vi "trackingNotification_Create.vi"(8 "error in (no error)":errorcluster, 9 "dim":i32, 10 "index":i32, 11 "reference in":refnum<class "trackingNotification.lvclass">) -> (0 "error out":errorcluster, 3 "reference out":refnum<class "trackingNotification.lvclass">)   [LabVIEW 2015, in "trackingNotification.lvclass"]
doc: "Constructor."
uses:
  trackingNotification.lvclass
  <vilib>/addons/_AddQ/G#Object/utils/G#Object_CreateMethod.ctl
  <vilib>/addons/_AddQ/G#Object/G#Object.lvclass
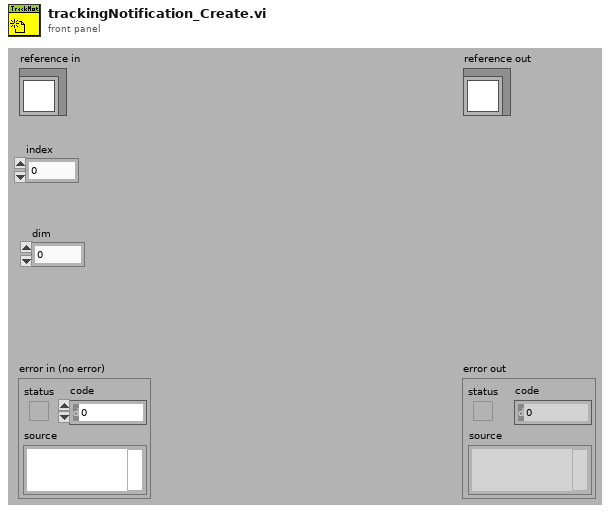
[diagram p1: front panel]
types:
  T1 = typedef "G#Object.lvclass/G#Object_CreateMethod.ctl" = enum16{"Create", "Create or look up existing", "Look up existing"}
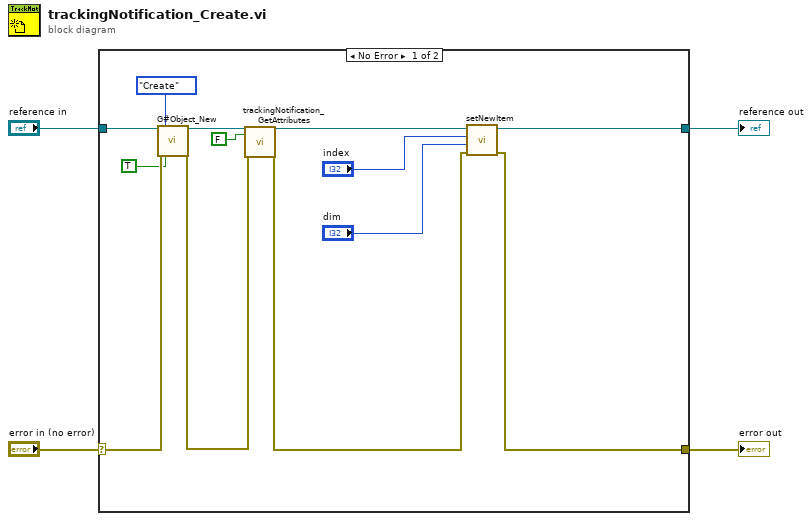
[diagram p0: block diagram]
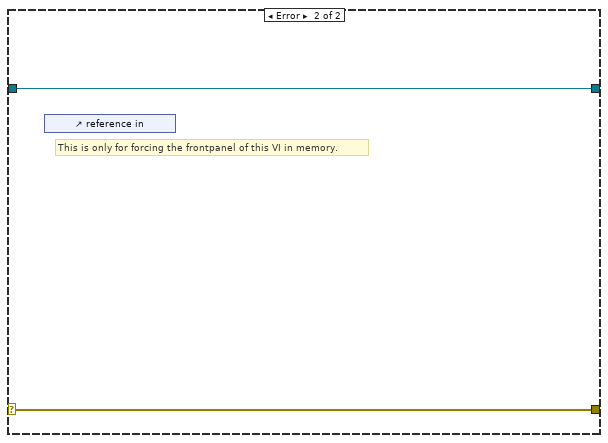
[diagram p2: hidden frame]
diagram:
  n1 = case shown="No Error" "error in (no error)" {
    selector: "error in (no error)" -> [w16 w19]
    tunnel: [w9 w19] -> w3
    tunnel: [w7 w18] -> w1
    tunnel: "reference in" -> [w17 w18]
    frame No Error {
      n2 = call <vilib>:"G#Object_New.vi"("reference in"=w17, "error in (no error)"=w16, "create method"=G#Object_CreateMethod."Create", "user counter (T)?"=TRUE ("User Counter")) -> ("reference out"=w14:refnum<class "trackingNotification.lvclass">, "error out"=w13:errorcluster)  [unwired: 13 in, 1 out]
      n3 = call "trackingNotification_GetAttributes.vi"("reference in"=w14, "return data? (T)"=FALSE ("return data"), "error in (no error)"=w13) -> ("reference out"=w8:refnum<class "trackingNotification.lvclass">, "error out"=w10:errorcluster)  [unwired: 13 in, 2 out]
      n4 = call "setNewItem.vi"("error in (no error)"=w10, "dim"="dim", "index"="index", "reference in"=w8) -> ("error out"=w9:errorcluster, "reference out"=w7:refnum<class "trackingNotification.lvclass">)  [unwired: 6 in]
    }
    frame Error {
      # "This is only for forcing the frontpanel of this VI in memory."
      n5 = control-ref of="reference in"() -> ()  [unwired: 1 out]
    }
  }
  "error out" <- w3
  "reference out" <- w1
